vi "DebugTestDevice.vi"() -> ()   [LabVIEW 2013]
uses:
  BaseDriver/BaseDriver.lvclass
  Point Grey Camera/Point Grey Camera.lvclass
panel:
  out "Application:Command Line Arguments":string[](array[string])
  out "error out 2":errorcluster
  out "specific class reference 2":refnum<class "BaseDriver.lvclass">
  in  "appended path 4":path=path "C:/GEECS/Developers Version/builds/Device builds/Copy of DebugDevice/DebugDevice.exe/Device Driver/Point Grey Camera/Point Grey Camera.lvclass"
  out "appended path 2":path
  out "appended path":path
  out "class path":path
  out "specific class reference":refnum<class "BaseDriver.lvclass">
  out "error out":errorcluster
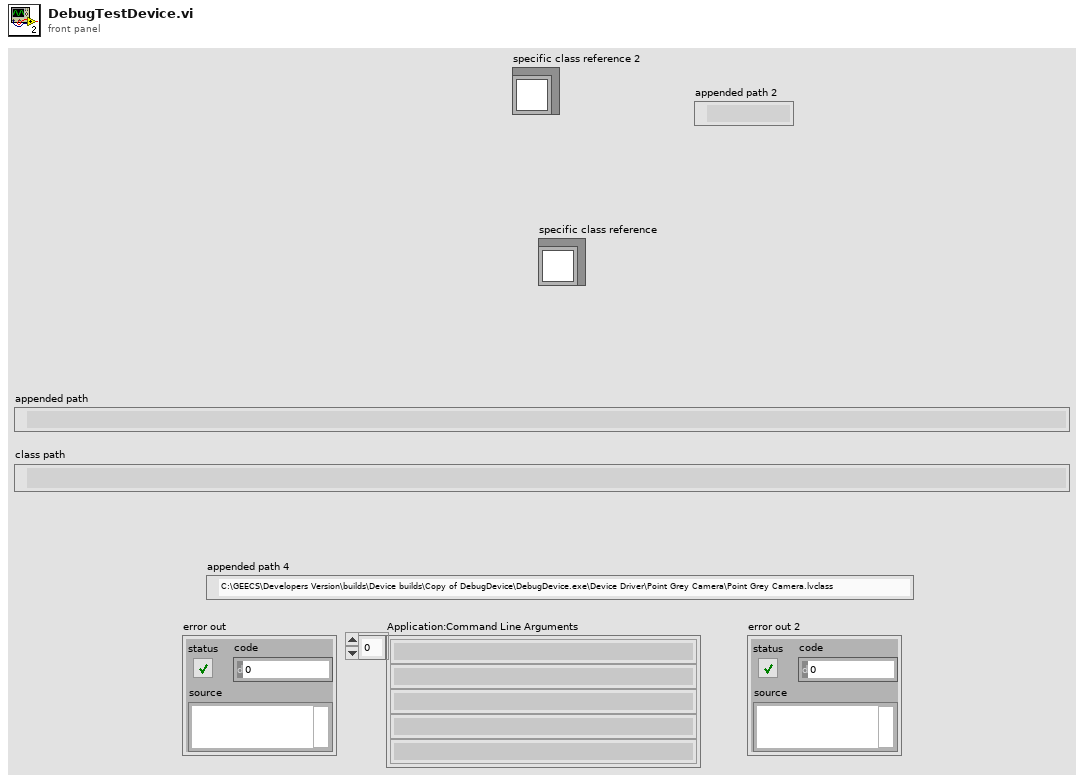
[diagram p1: front panel]
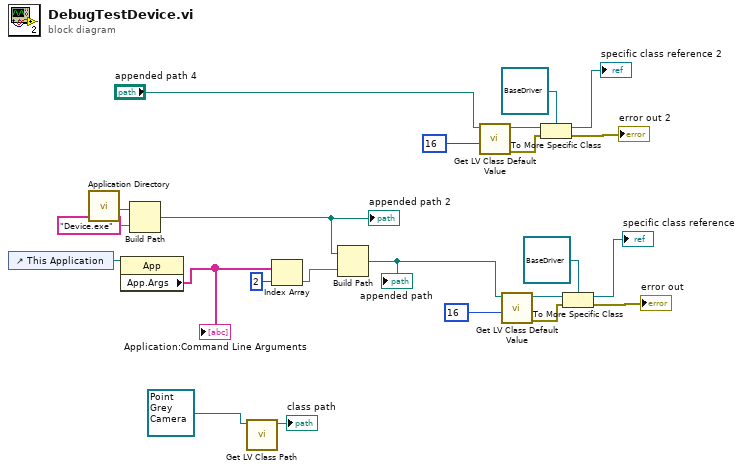
[diagram p0: block diagram]
diagram:
  n1 = control-ref of="This Application"() -> (w21:refnum<vi>)
  n2 = call <vilib>:"Application Directory.vi"() -> ("Application Directory"=w23:path)
  n3 = property class="App"(reference=w21) -> ("App.Args"=w20:string[])  [unwired: 1 in, 2 out]
  "Application:Command Line Arguments" <- w20
  n4 = Build Path(base path=w23, name or relative path="Device.exe") -> (appended path=w19:path)
  "appended path 2" <- w19
  n5 = call <vilib>:"Get LV Class Path.vi"("object"=refnum<class "Point Grey Camera.lvclass"> refnum ("Point Grey Camera.lvclass")) -> ("class path"=→"class path":path)  [unwired: 9 in, 1 out]
  n6 = Index Array(array=w20, index=2) -> (element=w18:string)
  n7 = Build Path(base path=w19, name or relative path=w18) -> (appended path=w13:path)
  "appended path" <- w13
  n8 = call <vilib>:"Get LV Class Default Value.vi"("options"=u32 16, "class path"="appended path 4") -> ("error out"=w2:errorcluster, "object"=w3:refnum<class>)  [unwired: 8 in]
  n9 = call <vilib>:"Get LV Class Default Value.vi"("options"=u32 16, "class path"=w13) -> ("error out"=w15:errorcluster, "object"=w14:refnum<class>)  [unwired: 8 in]
  n10 = To More Specific Class(target class=refnum<class "BaseDriver.lvclass"> refnum ("Driver"), reference=w3, error in=w2) -> (specific class reference=→"specific class reference 2":refnum<class "BaseDriver.lvclass">, error out=→"error out 2":errorcluster)
  n11 = To More Specific Class(target class=refnum<class "BaseDriver.lvclass"> refnum ("Driver"), reference=w14, error in=w15) -> (specific class reference=→"specific class reference":refnum<class "BaseDriver.lvclass">, error out=→"error out":errorcluster)
